vi "Initialize.vi"(8 "error in (no error)":errorcluster, 10 "Parameters in":refnum<class "Abstract Init Parameters.lvclass">=refnum, 11 "Abstract Switch Consumer in":refnum<class "Abstract Switch Consumer.lvclass">=refnum) -> (0 "error out":errorcluster, 3 "Abstract Switch Consumer out":refnum<class "Abstract Switch Consumer.lvclass">)   [LabVIEW 2019]
uses:
  Abstract Switch Init Parameters/Abstract Switch Init Parameters.lvclass
  Abstract Switch Consumer.lvclass
  Parameters/Abstract Init Parameters/Abstract Init Parameters.lvclass
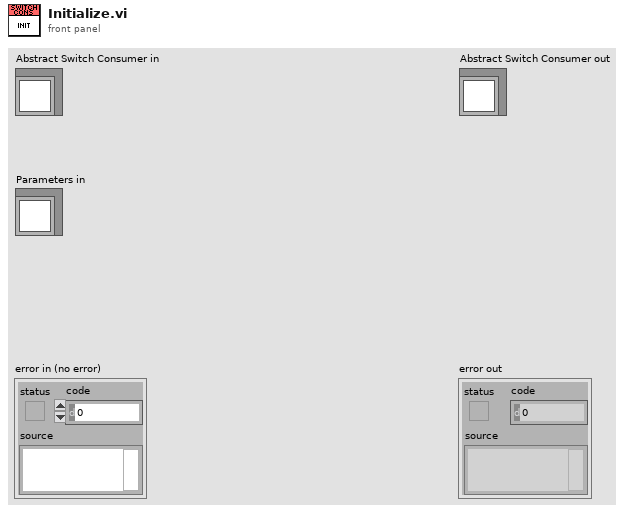
[diagram p1: front panel]
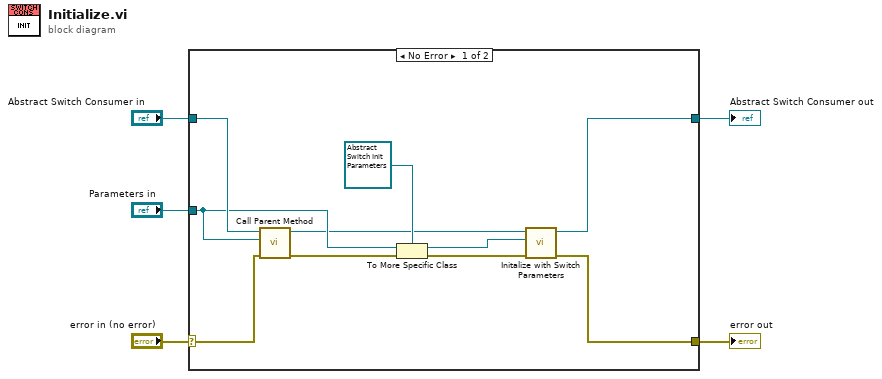
[diagram p0: block diagram]
diagram:
  n1 = case shown="No Error" "error in (no error)" {
    selector: "error in (no error)" -> [w11 w17]
    tunnel: [w6 w17] -> w4
    tunnel: [w8 w16] -> w3
    tunnel: "Abstract Switch Consumer in" -> [w13 w16]
    tunnel: "Parameters in" -> [w12 _]
    frame No Error {
      n2 = call-parent "Call Parent Method"("error in (no error)"=w11, "Parameters in"=w12, "Abstract Consumer in"=w13) -> ("error out"=w15:errorcluster, "Abstract Consumer out"=w9:refnum<class "Abstract Switch Consumer.lvclass">)  [unwired: 7 in]
      n3 = To More Specific Class(target class=refnum<class "Abstract Switch Init Parameters.lvclass"> refnum ("Message Queue Library.lvlib:Abstract Switch Init Parameters.lvclass"), reference=w12, error in=w15) -> (specific class reference=w10:refnum<class "Abstract Switch Init Parameters.lvclass">, error out=w7:errorcluster)
      n4 = call-dynamic "Initalize with Switch Parameters.vi"("error in (no error)"=w7, "Switch Parameters in"=w10, "Abstract Switch Consumer in"=w9) -> ("error out"=w6:errorcluster, "Abstract Switch Consumer out"=w8:refnum<class "Abstract Switch Consumer.lvclass">)  [unwired: 7 in]
    }
    frame Error {
    }
  }
  "error out" <- w4
  "Abstract Switch Consumer out" <- w3
